vi "GetSystemError.vi"(8 "error in (no error)":errorcluster, 11 "Retval":i32) -> (0 "error out":errorcluster)   [LabVIEW 2017]
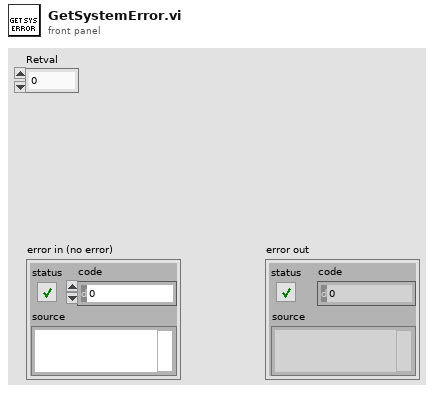
[diagram p1: front panel]
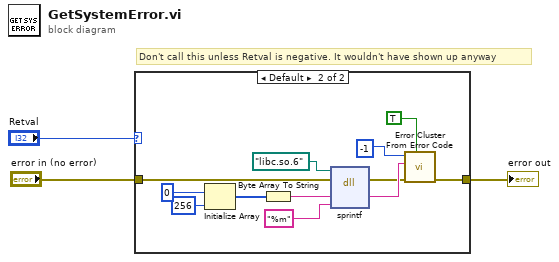
[diagram p0: block diagram]
diagram:
  # "Don't call this unless Retval is negative. It wouldn't have shown up anyway"
  n1 = case shown="Default" "Retval" {
    tunnel: "error in (no error)" -> [w4 w10]
    tunnel: [w4 w6] -> w2
    frame 0.. {
      # "Retval is 0 or positive"
    }
    frame Default {
      n2 = Initialize Array(u8 0, 256 ("dimension size")) -> (w13:u8[])
      n3 = Byte Array To String(unsigned byte array=w13) -> (string=w12:string)
      n4 = dll-call lib="?" fn="sprintf"(path in=path "libc.so.6", error in=w10, "str"=w12, "format"="%m" ("str")) -> (error out=w7:errorcluster, "str"=w8:string)  [unwired: 3 in, 1 out]
      n5 = call <vilib>:"Error Cluster From Error Code.vi"("show call chain? (False)"=TRUE, "error in (no error)"=w7, "error message (\"\")"=w8, "error code (0)"=-1) -> ("error out"=w6:errorcluster)  [unwired: 5 in]
    }
  }
  "error out" <- w2
